vi "fitGaussian.vi"(1 "initial parameters":dbl[](array[numeric])=[0.0, 1.0, 1.0, 1.0], 2 "X":dbl[](array[numeric]), 3 "Y":dbl[](array[numeric])) -> (0 "x0,sigma,bg,amplitude":dbl[](array[numeric]))   [LabVIEW 2017]
uses:
  <vilib>/gmath/NumericalOptimization/Nonlinear Curve Fit LM formula string.vi
  <vilib>/gmath/NI_Gmath.lvlib
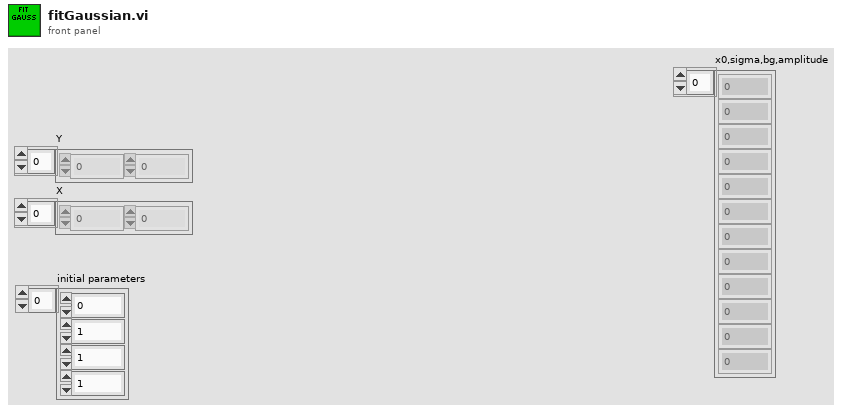
[diagram p1: front panel]
types:
  T1 = cluster{"model":string, "Parameters":string[], "x":string}
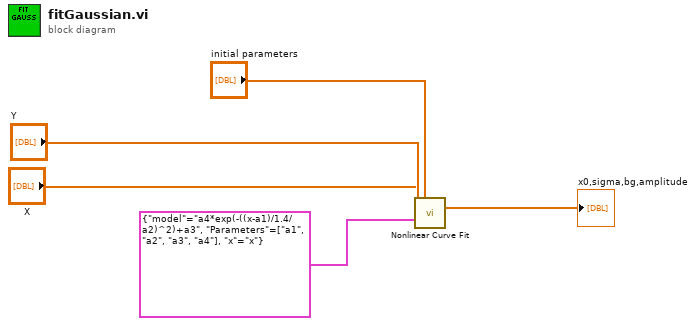
[diagram p0: block diagram]
diagram:
  n1 = call-poly <vilib>:"Nonlinear Curve Fit.vi"("Y"="Y", "initial parameters"="initial parameters", "X"="X", "model description"=T1 {"model"="a4*exp(-((x-a1)/1.4/a2)^2)+a3", "Parameters"=["a1", "a2", "a3", "a4"], "x"="x"}) -> ("best fit parameters"=→"x0,sigma,bg,amplitude":dbl[])  [unwired: 7 in, 4 out]
